vi "Productos inventario coffee.vi"(8 "error in (no error)":errorcluster, 10 "Productos inventario":i32, 11 "coffe actor in":refnum<class "coffe actor.lvclass">) -> (0 "error out":errorcluster, 3 "coffe actor out":refnum<class "coffe actor.lvclass">)   [LabVIEW 2020, in "coffe actor.lvlib" / "coffe actor.lvclass"]
uses:
  coffe actor.lvclass
  coffe actor.lvclass/coffe actor.ctl
  <vilib>/Utility/config.llb/Read Key (Double).vi
  <vilib>/Utility/config.llb/Write Key (String).vi
  <vilib>/Utility/config.llb/Read Key (String).vi
  <vilib>/Utility/config.llb/NI_LVConfig.lvlib
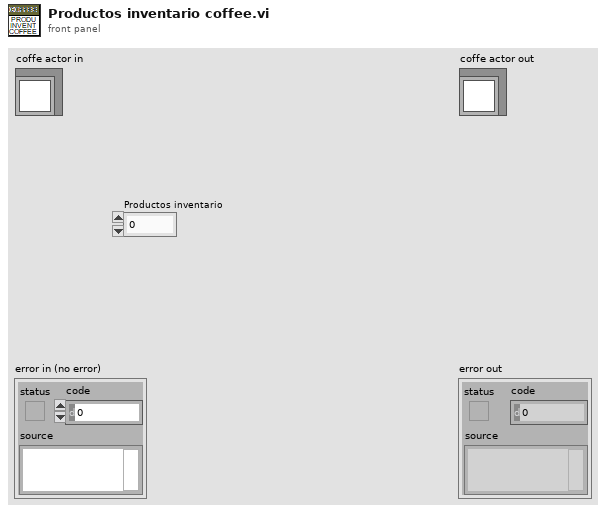
[diagram p1: front panel]
types:
  T1 = typedef "NI_LVConfig.lvlib/Config Data RefNum.ctl" = refnum<k1>
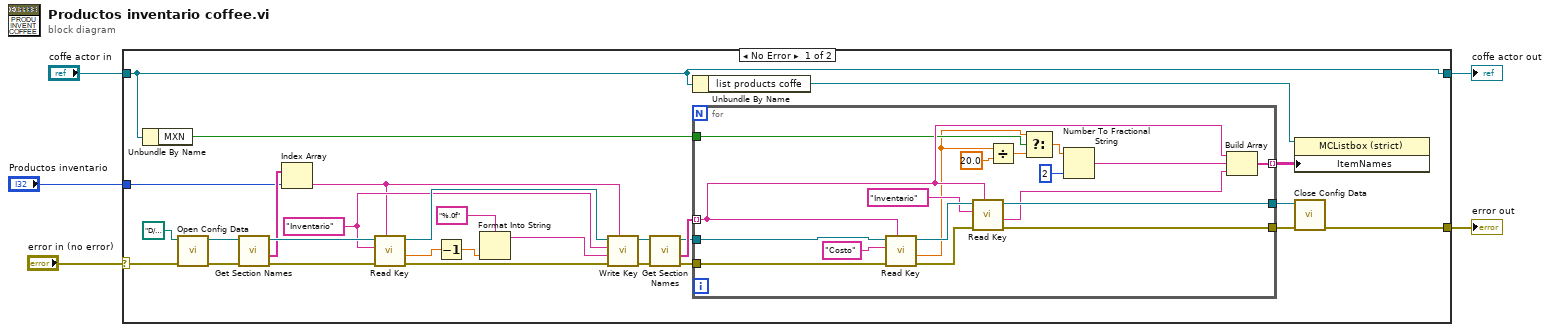
[diagram p0: block diagram]
diagram:
  n1 = case shown="No Error" "error in (no error)" {
    selector: "error in (no error)" -> [w9 w53]
    tunnel: [w8 w53] -> w4
    tunnel: [w7 w52] -> w2
    tunnel: "coffe actor in" -> [w7 w52]
    tunnel: "Productos inventario" -> [w6 _]
    frame No Error {
      w22 = "Inventario" ("key")
      n2 = Unbundle By Name(w7) -> ("MXN"=w11:bool)
      n3 = call <vilib>:"Open Config Data.vi"("error in (no error)"=w9, "configuration file path"=path "D:/fork/Maquina-Expendedora/maquina/coffe actor.ini") -> ("error out"=w33:errorcluster, "refnum"=w32:T1)  [unwired: 7 in, 1 out]
      n4 = call <vilib>:"Get Section Names.vi"("error in (no error)"=w33, "refnum"=w32) -> ("error out"=w27:errorcluster, "section names"=w29:string[], "refnum out"=w31:T1)  [unwired: 7 in]
      n5 = Index Array "Index Array"(array=w29, index=w6) -> (element=w10:string)
      n6 = call-poly <vilib>:"Read Key.vi"("section"=w10, "error in (no error)"=w27, "key"=w22, "refnum"=w31) -> ("error out"=w21:errorcluster, "value"=w28:dbl, "refnum out"=w23:T1)  [unwired: 4 in, 1 out]
      n7 = Decrement(x=w28) -> (x-1=w25:dbl)
      n8 = Format Into String "Format Into String"(format string="%.0f", w25) -> (resulting string=w24:string)  [unwired: 2 in, 1 out]
      n9 = call-poly <vilib>:"Write Key.vi"("section"=w10, "error in (no error)"=w21, "value"=w24, "key"=w22, "refnum"=w23) -> ("error out"=w20:errorcluster, "refnum out"=w19:T1)  [unwired: 4 in, 1 out]
      n10 = call <vilib>:"Get Section Names.vi"("error in (no error)"=w20, "refnum"=w19) -> ("error out"=w18:errorcluster, "section names"=w17:string[], "refnum out"=w16:T1)  [unwired: 7 in]
      n11 = Unbundle By Name(w7) -> ("list products coffe"=w12:refnum<vi>)
      n12 = for {
        tunnel: w16 -> [w51]
        tunnel: w18 -> [w50]
        tunnel: [w47] -> w15
        tunnel: [w46] -> w14
        tunnel: w11 -> [w38]
        tunnel: w17 -> [w43] mode=indexing
        tunnel: [w41] -> w13 mode=indexing
        n13 = call-poly <vilib>:"Read Key.vi"("section"=w43, "error in (no error)"=w50, "key"="Costo", "refnum"=w51) -> ("error out"=w49:errorcluster, "value"=w36:dbl, "refnum out"=w48:T1)  [unwired: 4 in, 1 out]
        n14 = call-poly <vilib>:"Read Key.vi"("section"=w43, "error in (no error)"=w49, "key"="Inventario", "refnum"=w48) -> ("error out"=w47:errorcluster, "value"=w42:string, "refnum out"=w46:T1)  [unwired: 4 in, 1 out]
        n15 = Divide(x=w36, y=20.0) -> (x/y=w34:dbl)
        n16 = Select(t=w36, s=w38, f=w34) -> (s? t:f=w37:dbl)
        n17 = Number To Fractional String(number=w37, precision (6)=i16 2) -> (F-format string=w40:string)  [unwired: 2 in]
        n18 = Build Array(w43, w40, w42) -> (w41:string[])
      }
      n19 = property class="MCListbox (strict)"(reference=w12, "ItemNames"=w13) -> ()  [unwired: 1 in, 2 out]
      n20 = call <vilib>:"Close Config Data.vi"("error in (no error)"=w15, "refnum"=w14) -> ("error out"=w8:errorcluster)  [unwired: 8 in, 1 out]
    }
    frame Error {
    }
  }
  "error out" <- w4
  "coffe actor out" <- w2
